vi "Configure Timebase.vi"(7 "Record Length (10000)":u32=10000 caption="Record Length (10000s)", 8 "error in (no error)":errorcluster, 9 "Position (0.0 s)":dbl=50.0, 10 "horizontal scale (t/div)":ext(ring)=4e-7 items=["400ns/div", "1µs/div", "2µs/div", "4µs/div", "10µs/div", "20µs/div"], 11 "VISA resource name":refnum<visa-resource-name>) -> (0 "error out":errorcluster, 3 "VISA resource name out":refnum<visa-resource-name>)   [LabVIEW 2011, in "Tektronix 7000 Series.lvlib"]
doc: "Configures the timebase and horizontal properties of an oscilloscope."
uses:
  Tektronix 7000 Series.lvlib
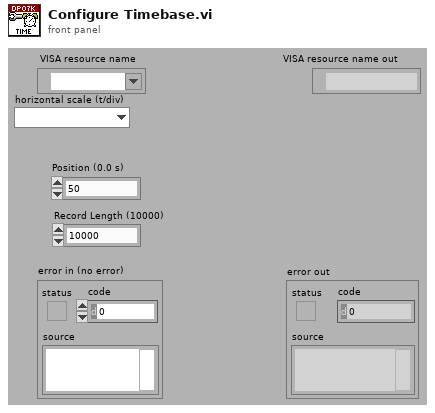
[diagram p1: front panel]
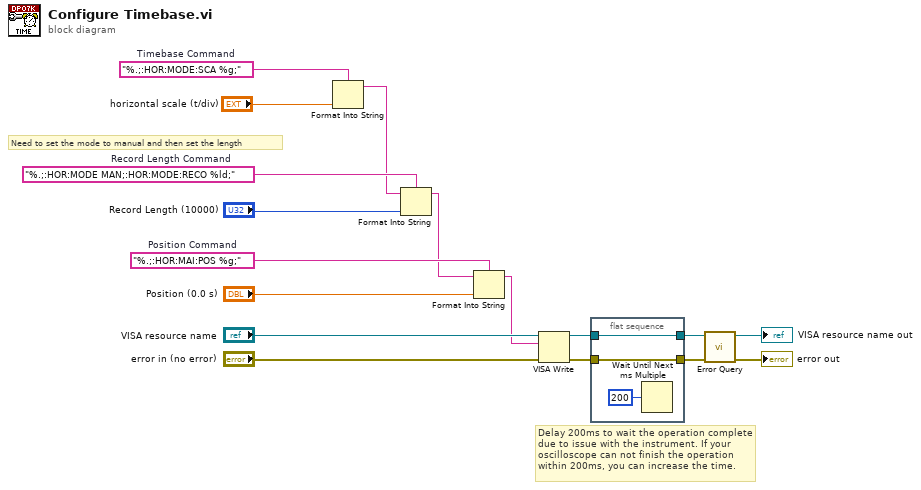
[diagram p0: block diagram]
diagram:
  w14 = "%.;:HOR:MODE MAN;:HOR:MODE:RECO %ld;"  # Record Length Command
  w16 = "%.;:HOR:MAI:POS %g;"  # Position Command
  w17 = "%.;:HOR:MODE:SCA %g;"  # Timebase Command
  # "Need to set the mode to manual and then set the length"
  # "Delay 200ms to wait the operation complete due to issue with the instrument. If your oscilloscope can not finish the operation within 200ms, you can increase the time."
  n1 = Format Into String(format string=w17, "horizontal scale (t/div)") -> (resulting string=w3:string)  [unwired: 2 in, 1 out]
  n2 = Format Into String(format string=w14, initial string=w3, "Record Length (10000)") -> (resulting string=w2:string)  [unwired: 1 in, 1 out]
  n3 = Format Into String(format string=w16, initial string=w2, "Position (0.0 s)") -> (resulting string=w4:string)  [unwired: 1 in, 1 out]
  n4 = VISA Write(VISA resource name="VISA resource name", write buffer=w4, error in (no error)="error in (no error)") -> (VISA resource name out=w11:refnum<visa-resource-name>, error out=w10:errorcluster)  [unwired: 1 out]
  n5 = flat-sequence {
    tunnel: w11 -> [w19]
    tunnel: [w19] -> w8
    tunnel: w10 -> [w18]
    tunnel: [w18] -> w9
    frame #0 {
      n6 = Wait Until Next ms Multiple(millisecond multiple=u32 200) -> ()  [unwired: 1 out]
    }
  }
  n7 = call "Error Query.vi"("error in (no error)"=w9, "VISA resource name"=w8) -> ("error out"=→"error out":errorcluster, "VISA resource name out"=→"VISA resource name out":refnum<visa-resource-name>)  [unwired: 6 in, 2 out]
